vi "NISE.Get Generic Property (Core).vi"(0 "SLSC Interface in":refnum<class "SLSC Interface.lvclass">, 1 "property type":T1, 5 "resources":string, 7 "property":refnum<k21>, 11 "error in (no error)":errorcluster) -> (4 "SLSC Interface out":refnum<class "SLSC Interface.lvclass">, 10 "property value":variant, 15 "error out":errorcluster)   [LabVIEW 2016, in "SLSC Interface.lvclass"]
uses:
  SLSC Interface.lvclass
  Property Type.ctl
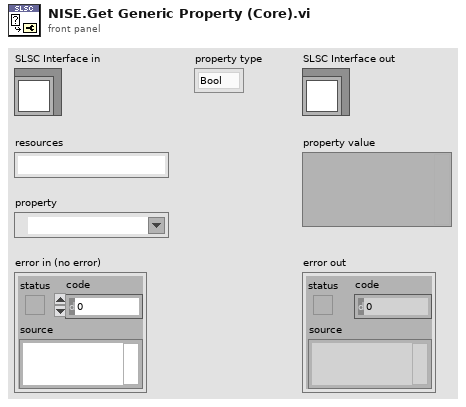
[diagram p1: front panel]
types:
  T1 = typedef "SLSC Interface.lvclass/Property Type.ctl" = enum16{"Bool", "DBL", "I32", "I64", "String", "U32", "U64", "1D Bool", "1D DBL", "1D I32", "1D I64", "1D String", "1D U32", "1D U64"}
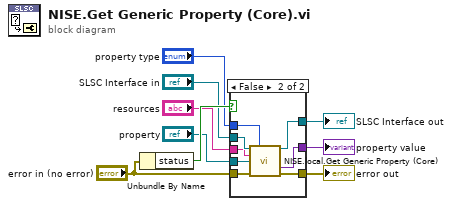
[diagram p0: block diagram]
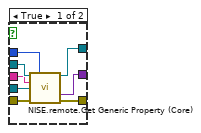
[diagram p2: hidden frame]
diagram:
  n1 = Unbundle By Name("error in (no error)") -> ("status"=w9:bool)
  n2 = case shown="False" w9 {
    tunnel: "SLSC Interface in" -> [w17 w25]
    tunnel: "property type" -> [w16 w24]
    tunnel: [w15 w23] -> w6
    tunnel: "resources" -> [w14 w22]
    tunnel: "property" -> [w13 w21]
    tunnel: [w12 w20] -> w3
    tunnel: "error in (no error)" -> [w11 w19]
    tunnel: [w10 w18] -> w1
    frame True {
      n3 = call "NISE.remote.Get Generic Property (Core).vi"("SLSC Remote in"=w17, "property type"=w16, "resources"=w14, "property"=w13, "error in (no error)"=w11) -> ("SLSC Remote out"=w15:refnum<class "SLSC Interface.lvclass">, "property value"=w12:variant, "error out"=w10:errorcluster)  [unwired: 8 in]
    }
    frame False {
      n4 = call "NISE.local.Get Generic Property (Core).vi"("SLSC Local in"=w25, "property type"=w24, "resources"=w22, "property"=w21, "error in (no error)"=w19) -> ("SLSC Local out"=w23:refnum<class "SLSC Interface.lvclass">, "property value"=w20:variant, "error out"=w18:errorcluster)  [unwired: 8 in]
    }
  }
  "error out" <- w1
  "SLSC Interface out" <- w6
  "property value" <- w3
